vi "Text2012.vi"   [LabVIEW 2013]
uses:
  <vilib>/Heliosphere Research LLC/Advanced Plotting Toolkit/api_annotations/TextProperties.ctl
  <vilib>/Heliosphere Research LLC/Advanced Plotting Toolkit/properties/Text.ctl
  <vilib>/Heliosphere Research LLC/Advanced Plotting Toolkit/typedefs/PlotColor.ctl
  <vilib>/Heliosphere Research LLC/Advanced Plotting Toolkit/properties/Text_FontSize.ctl
  <vilib>/Heliosphere Research LLC/Advanced Plotting Toolkit/properties/Text_FontStyle.ctl
  <vilib>/Heliosphere Research LLC/Advanced Plotting Toolkit/properties/Display.ctl
  <vilib>/Heliosphere Research LLC/Advanced Plotting Toolkit/Advanced Plotting Toolkit.lvlib
types:
  T1 = typedef "Advanced Plotting Toolkit.lvlib/TextProperties.ctl" = cluster{"Text":T2, "Display":T6}
  T2 = typedef "Advanced Plotting Toolkit.lvlib/Text.ctl" = cluster{"Color":T3, "Background Color":T3, "Font Size (points)":T4, "Font Style":T5, "Rotation Angle":dbl}
  T3 = typedef "Advanced Plotting Toolkit.lvlib/PlotColor.ctl" = u32
  T4 = typedef "Advanced Plotting Toolkit.lvlib/Text_FontSize.ctl" = i32
  T5 = typedef "Advanced Plotting Toolkit.lvlib/Text_FontStyle.ctl" = enum16{"Automatic", "Normal", "Italic", "Bold"}
  T6 = typedef "Advanced Plotting Toolkit.lvlib/Display.ctl" = cluster{"Alpha":dbl, "Z Order":dbl}
  T7 = typedef "Advanced Plotting Toolkit.lvlib/PlotID.ctl" = i32
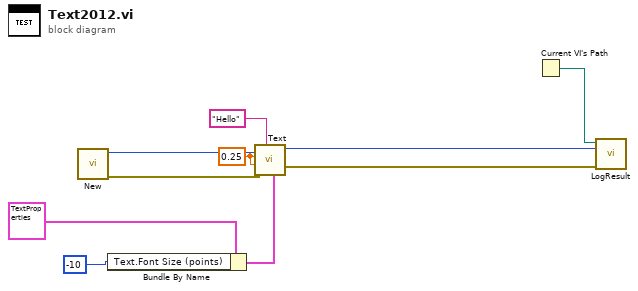
[diagram p0: block diagram]
diagram:
  w9 = 0.25 ("X Position")
  n1 = call <vilib>:"New.vi"() -> ("error out"=w6:errorcluster, "Plot ID"=w7:T7)  [unwired: 10 in]
  n2 = Bundle By Name(cluster=T1 {"Text"={"Color"=2147483647, "Background Color"=2147483647, "Font Size (points)"=0, "Font Style"=enum."Automatic", "Rotation Angle"=nan}, "Display"={"Alpha"=nan, "Z Order"=nan}} ("Text Properties"), "Text.Font Size (points)"=-10) -> (w2:T1)
  n3 = call <vilib>:"Text.vi"("Properties"=w2, "Text"="Hello", "error in (no error)"=w6, "Y Position"=w9, "X Position"=w9, "Plot ID"=w7) -> ("error out"=w4:errorcluster, "Plot ID Out"=w5:T7)  [unwired: 4 in]
  n4 = Current VI's Path() -> (path=w10:path)
  n5 = call "LogResult.vi"("Test Result"=w4, "Test Artifact"=w5, "VI Path"=w10) -> ()  [unwired: 9 in]
